vi "Rewire Do.vi"(8 "error in (no error)":errorcluster, 11 "Replace":refnum<vi>) -> (0 "error out":errorcluster, 3 "done?":bool)   [LabVIEW 2020, in "Message Maker.lvlib"]
uses:
  Message Maker.lvlib
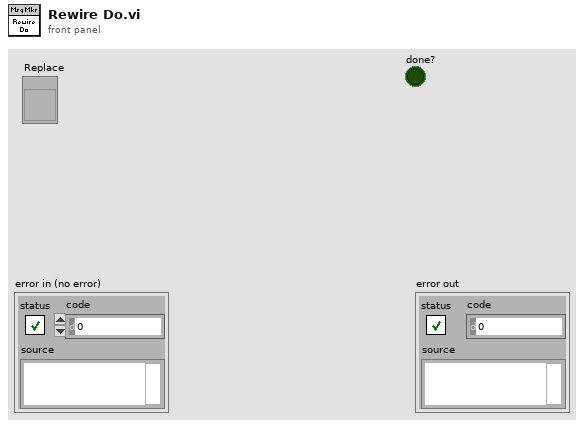
[diagram p1: front panel]
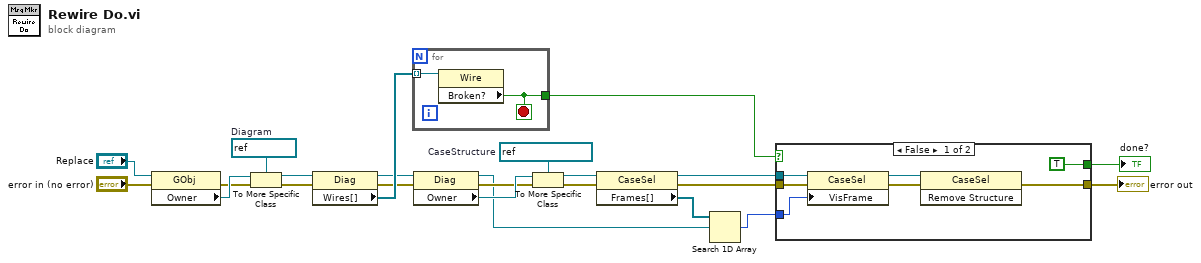
[diagram p0: block diagram]
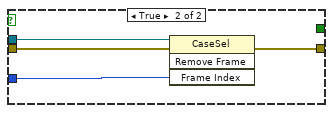
[diagram p2: hidden frame]
diagram:
  w14 = refnum<vi> refnum  # CaseStructure
  w21 = refnum<vi> refnum  # Diagram
  n1 = property class="GObj"(reference="Replace", error in="error in (no error)") -> (error out=w20:errorcluster, "Owner"=w22:refnum<vi>)  [unwired: 1 out]
  n2 = To More Specific Class(target class=w21, reference=w22, error in=w20) -> (specific class reference=w16:refnum<vi>, error out=w15:errorcluster)
  n3 = property class="Diag"(reference=w16, error in=w15) -> (reference out=w13:refnum<vi>, error out=w11:errorcluster, "Wires[]"=w17:refnum<vi>[])
  n4 = for {
    tunnel: w17 -> [w25] mode=indexing
    tunnel: [w24] -> w9
    stop <- w24 stop-if-true
    n5 = property class="Wire"(reference=w25) -> ("Broken?"=w24:bool)  [unwired: 1 in, 2 out]
  }
  n6 = property class="Diag"(reference=w13, error in=w11) -> (reference out=w5:refnum<vi>, error out=w10:errorcluster, "Owner"=w12:refnum<vi>)
  n7 = To More Specific Class(target class=w14, reference=w12, error in=w10) -> (specific class reference=w8:refnum<vi>, error out=w7:errorcluster)
  n8 = property class="CaseSel"(reference=w8, error in=w7) -> (reference out=w2:refnum<vi>, error out=w1:errorcluster, "Frames[]"=w6:refnum<vi>[])
  n9 = Search 1D Array(1D array=w6, element=w5) -> (index of element=w3:i32)  [unwired: 1 in]
  n10 = case shown="False" w9 {
    tunnel: [w32 w35] -> w18
    tunnel: w1 -> [w28 w34]
    tunnel: [TRUE _] -> w4
    tunnel: w2 -> [w30 w36]
    tunnel: w3 -> [w26 w33]
    frame False {
      n11 = property class="CaseSel"(reference=w30, error in=w28, "VisFrame"=w26) -> (reference out=w29:refnum<vi>, error out=w27:errorcluster)
      n12 = invoke class="CaseSel" method="Remove Structure"(reference=w29, error in=w27) -> (error out=w32:errorcluster)  [unwired: 1 in, 2 out]
    }
    frame True {
      n13 = invoke class="CaseSel" method="Remove Frame"(reference=w36, error in=w34, "Frame Index"=w33) -> (error out=w35:errorcluster)  [unwired: 1 in, 3 out]
    }
  }
  "error out" <- w18
  "done?" <- w4
